vi "Selection.vi"(8 "error in (no error)":errorcluster, 11 "TSP Class in":refnum<class "TSP Class.lvclass">) -> (0 "error out":errorcluster, 3 "TSP Class out":refnum<class "TSP Class.lvclass">)   [LabVIEW 2015, in "TSP Library.lvlib" / "TSP Class.lvclass"]
uses:
  TSP Class.lvclass
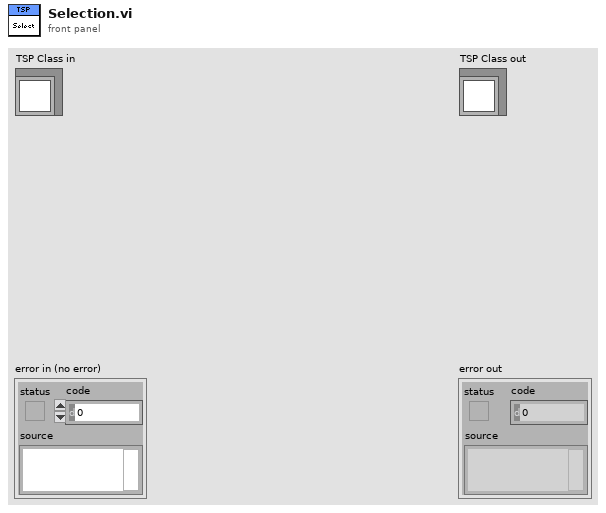
[diagram p1: front panel]
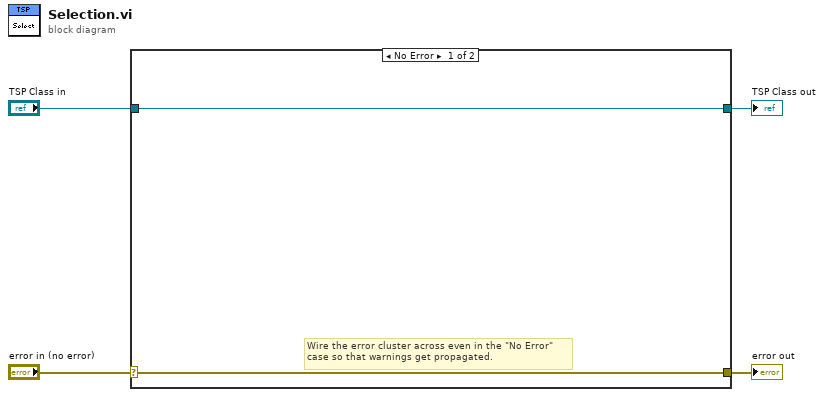
[diagram p0: block diagram]
diagram:
  n1 = case shown="No Error" "error in (no error)" {
    selector: "error in (no error)" -> [w5 w8]
    tunnel: [w5 w8] -> w3
    tunnel: [w6 w7] -> w1
    tunnel: "TSP Class in" -> [w6 w7]
    frame No Error {
      # "Wire the error cluster across even in the \"No Error\"\ncase so that warnings get propagated."
    }
    frame Error {
    }
  }
  "error out" <- w3
  "TSP Class out" <- w1
